vi "Results_Space_Analysis.vi"(0 "Table":string[][](table)) -> ()   [LabVIEW 2010]
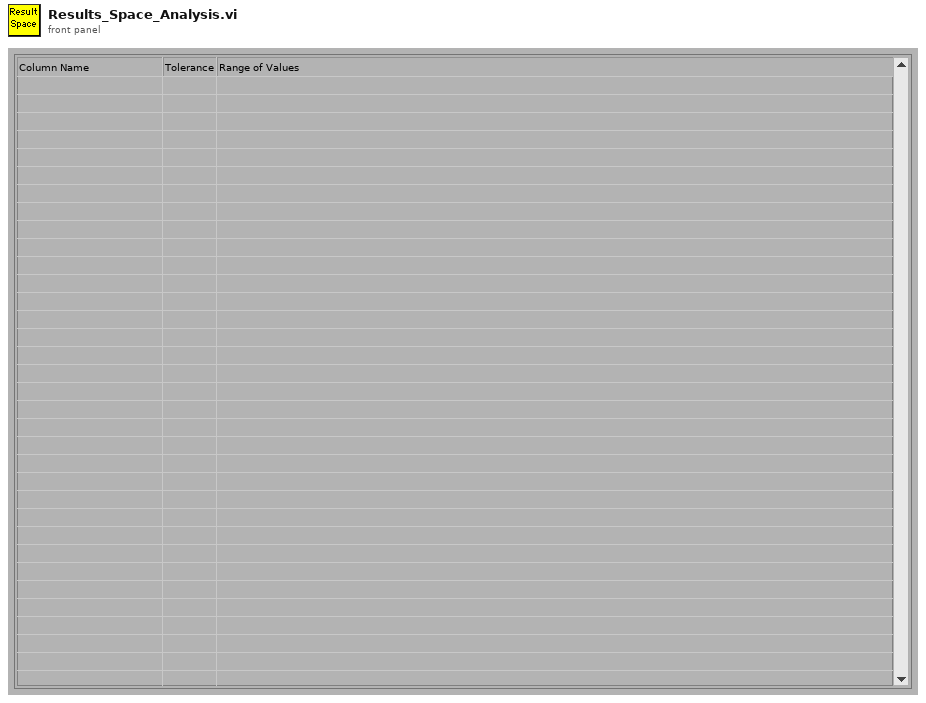
[diagram p1: front panel]
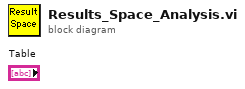
[diagram p0: block diagram]
diagram:
